vi "Dashboard Main.vi"() -> ()   [LabVIEW 2013]
uses:
  <vilib>/Rock Robotics/WPI/Camera/WPI_CameraSettings Read MJPG.ctl
  <vilib>/Rock Robotics/WPI/Camera/WPI_CameraImageSize.ctl
  <vilib>/Rock Robotics/WPI/Dashboard/WPI_DashboardLogging Global.vi
  <vilib>/vision/NI_Vision_Development_Module.lvlib
panel:
  out "Left":dbl(slide) scale=-1.0..1.0
  out "Right":dbl(slide) scale=-1.0..1.0
  out "Switch States":bool[](array[boolean])
  out "Catapult State":string
  out "Skeleton Detected":bool
  out "Right Triggered":bool
  out "Left Triggered":bool
  in  "Autonomous Mode":T1(ring)
  out "Right Speed":dbl(knob) scale=-11.0..11.0
  out "Left Speed":dbl(knob) scale=-11.0..11.0
  out "Teleop Time":dbl(slide) scale=0.0..150.0
  out "Right Power":dbl(slide) scale=-1.0..1.0
  out "Left Power":dbl(slide) scale=-1.0..1.0
  in  "Camera view range":dbl=33.5 format="%#_13g"
  out "Time Remaining":dbl(slide) scale=0.0..150.0
  in  "stop":bool
  out "Camera IP":string
  in  "DB Camera Config":bool
  out "Image Message":string="Timeout in Camera Communications"
  in  "Rec Mode":enum32{"Stop", "Record", "Playback"}(radio)
  out "Secondary Driver Camera":T2(plugin-control)
  out "Primary Driver Camera":T2(plugin-control)
  # "Primary Driver Side"
  # "Secondary Driver Side"
  # "TeleOperated"
  # "Autonomous"
  # "Checklist:\n1: DO WE HAVE A CHARGED BATTERY?\n2: Is the robot plugged in?\n3: Is the robot turned on?\n4: Are the ball(s) in the correct position?\n5: Set up Autonomous (One or Two balls?)"
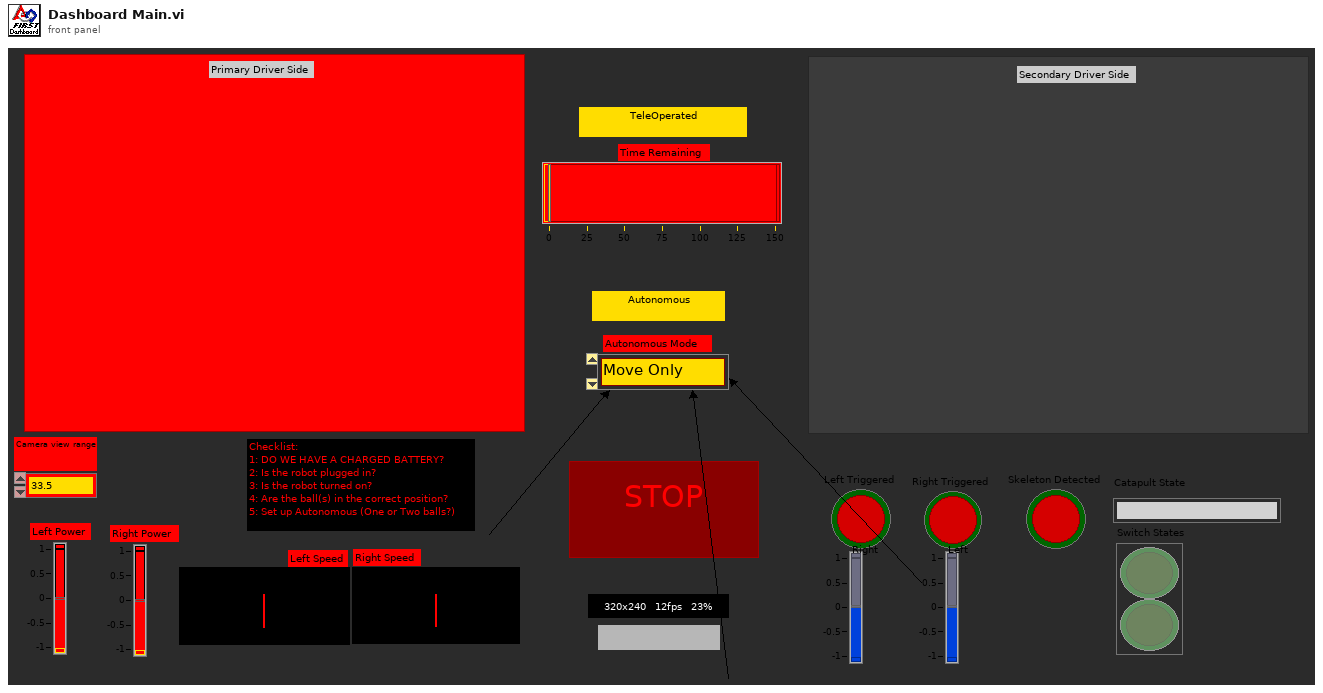
[diagram p1: front panel]
types:
  T1 = enum16{"Move Only", "One Ball", "Two Ball", "Three Ball", "Two Ball Hot", "One Ball Hot", "Nothing"}
  T2 = typedef "IMAQ Image.ctl" = refnum<image>
  T3 = typedef "Image Type" = u32
  T4 = cluster{"Left Power":dbl, "Right Power":dbl, "Shooter State":enum16{"Nothing", "Cocked", "Fire", "Load"}, "Loader State":enum16{"Loader Up", "Loader Down", "Ball In Possesion"}, "Auto Time":dbl, "Tele Time":dbl, "Driver":dbl, "Not Allowed":bool, "Right Speed":dbl, "Left Speed":dbl}
  T5 = cluster{"Digital Inputs":bool[], "Digital Outputs":bool[]}
  T6 = cluster{"Competition mode":bool, "Robot Link":bool, "Autonomous":bool, "Enabled":bool, "E-Stop":bool, "Simulated":bool, "TestMode":bool, "Docked Window":bool}
  T7 = typedef "Vector4.ctl" = cluster{"x":sgl, "y":sgl, "z":sgl, "w":sgl}
  T8 = typedef "SkeletonTrackState.ctl" = enum32{"NotTracked", "PositionOnly", "Tracked"}
  T9 = typedef "WPI_JoystickDeviceDataRaw.ctl" = cluster{"axis 1":i8, "axis 2":i8, "axis 3":i8, "axis 4":i8, "axis 5":i8, "axis 6":i8, "Buttons":u16}
  T10 = cluster{cluster{"Version String":string, "Number of Players":i8, "Flags":u32, "FloorClipPlane":T7, "Gravity Normal":cluster{"x":sgl, "y":sgl, "z":sgl}}, cluster{"TrackingState":u8[], "Overall Position":cluster{"x":sgl, "y":sgl, "z":sgl}, "Quality":u32, "TrackState":T8}, "Skeleton Vertices":cluster{"x":sgl, "y":sgl, "z":sgl}[], "Joystick":T9, "Joystick 2":T9, "Custom Data":string}
  T11 = typedef "WPI_CameraSettings Read MJPG.ctl" = cluster{"fps":i32, "compression":i32, "Image Size":T12}
  T12 = typedef "WPI_CameraImageSize.ctl" = enum16{"640x480", "320x240", "160x120"}
  T13 = cluster{"Left":i32, "Top":i32, "Right":i32, "Bottom":i32}
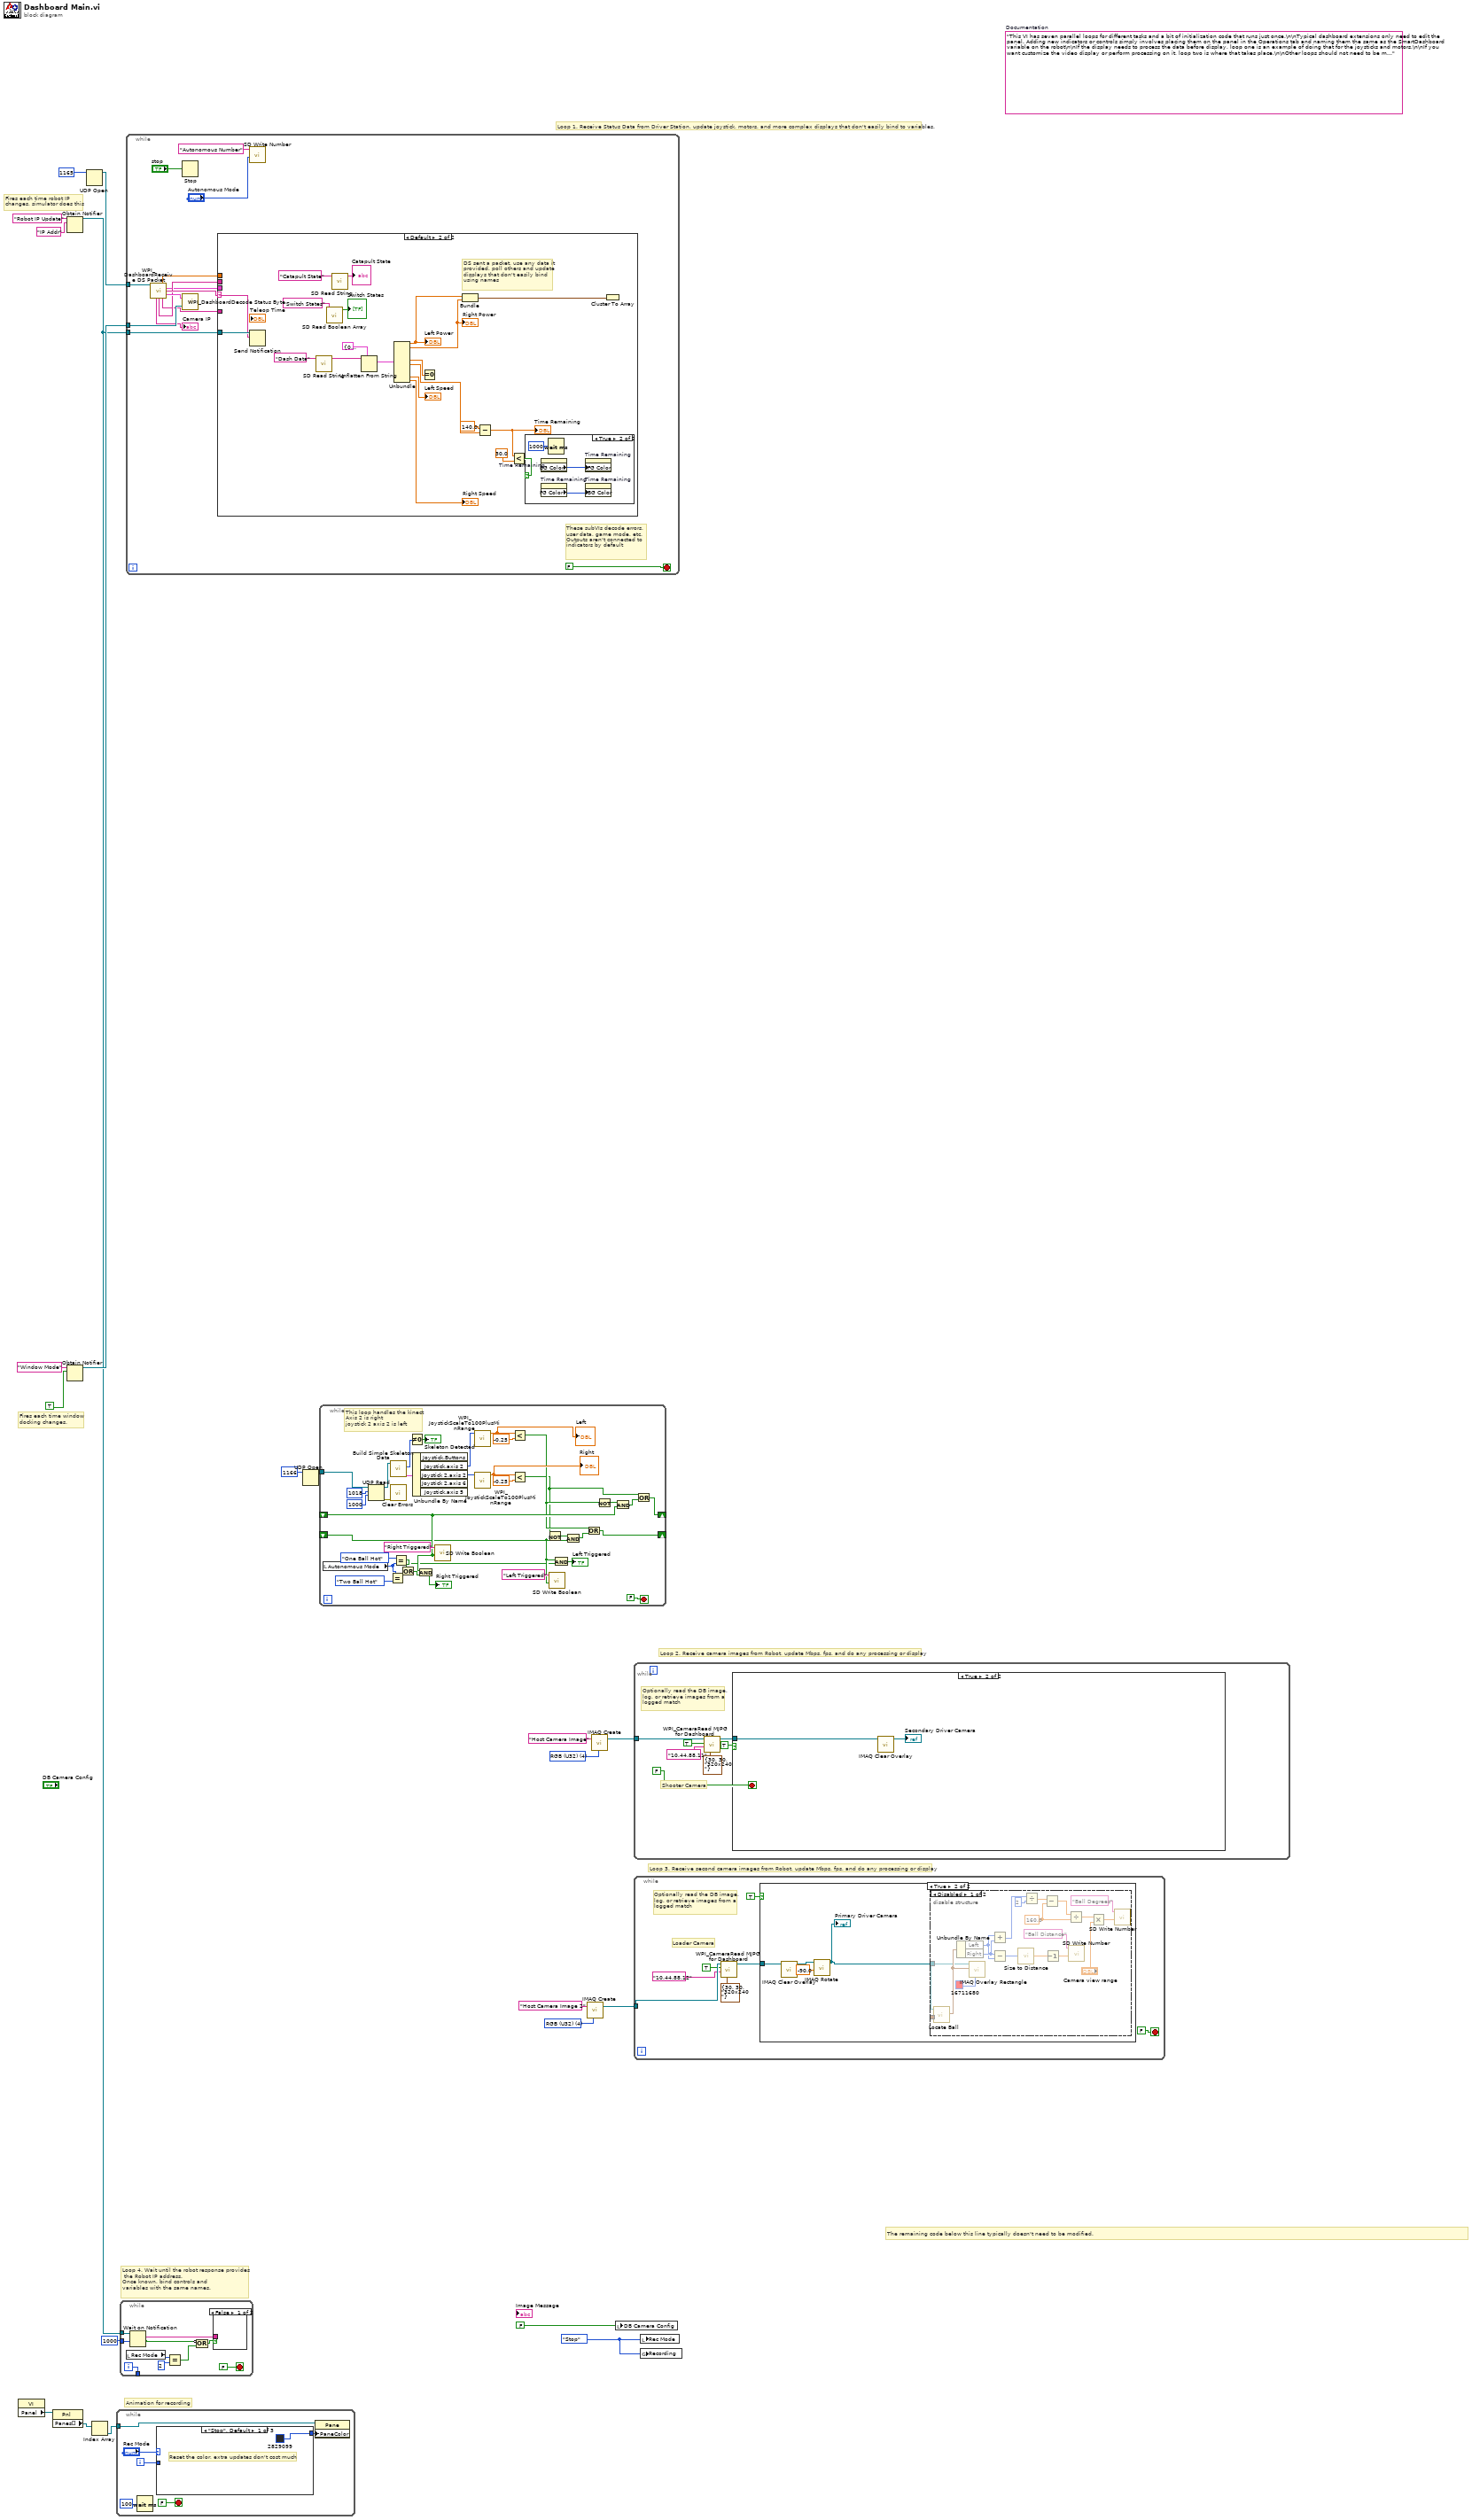
[diagram p0: block diagram]
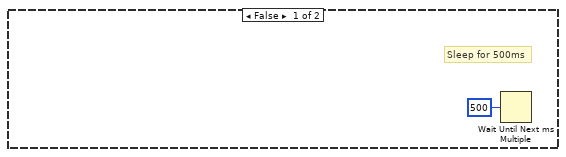
[diagram p2: hidden frame]
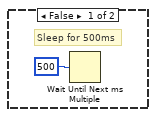
[diagram p3: hidden frame]
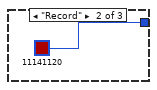
[diagram p5: hidden frame]
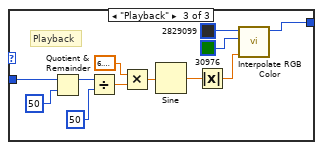
[diagram p6: hidden frame]
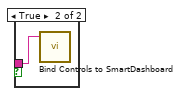
[diagram p7: hidden frame]
diagram:
  w5 = T3 4 items=["Grayscale (U8)", "Grayscale (I16)", "Grayscale (SGL)", "Complex (CSG)", "RGB (U32)", "HSL (U32)", "RGB (U64)"] ("Image Type")
  w6 = T3 4 items=["Grayscale (U8)", "Grayscale (I16)", "Grayscale (SGL)", "Complex (CSG)", "RGB (U32)", "HSL (U32)", "RGB (U64)"] ("Image Type")
  w10 = enum32{"Stop", "Record", "Playback"}."Stop" ("Rec Mode")
  (unwired) "This VI has seven parallel loops for different tasks and a bit of initialization code that runs just once.\n\nTypical dashboard extensions only need to edit the panel. Adding new indicators or controls simply involves placing them on the panel in the Operations tab and naming them the same as the SmartDashboard variable on the robot\n\nIf the display needs to process the data before display, loop one is an example of doing that for the joysticks and motors.\n\nIf you want customize the video display or perform processing on it, loop two is where that takes place.\n\nOther loops should not need to be modified. They are pretty standard, and document the task they perform."  # Documentation
  # "Loop 3. Receive second camera images from Robot, update Mbps, fps, and do any processing or display"
  # "Loop 2. Receive camera images from Robot, update Mbps, fps, and do any processing or display"
  # "Animation for recording"
  # "Fires each time robot IP\nchanges, simulator does this"
  # "Fires each time window\ndocking changes."
  # "The remaining code below this line typically doesn't need to be modified."
  # "Loop 4. Wait until the robot response provides\n the Robot IP address.\nOnce known, bind controls and\nvariables with the same names."
  # "Loop 1. Receive Status Data from Driver Station, update joystick, motors, and more complex displays that don't easily bind to variables."
  n1 = property class="VI"() -> ("Panel"=w14:refnum<vi>)  [unwired: 2 in, 2 out]
  n2 = property class="Pnl"(reference=w14) -> ("Panes[]"=w15:refnum<vi>[])  [unwired: 1 in, 2 out]
  n3 = Obtain Notifier(name (unnamed)="Robot IP Update", notification data type="IP Addr" ("name (unnamed)")) -> (notifier out=w9:refnum<notifier>)  [unwired: 2 in, 2 out]
  n4 = Obtain Notifier(name (unnamed)="Window Mode", notification data type=TRUE) -> (notifier out=w11:refnum<notifier>)  [unwired: 2 in, 2 out]
  n5 = UDP Open(11:u16 1165 ("port")) -> (port=w21:refnum<k16>)  [unwired: 2 in, 4 out]
  n6 = Index Array(array=w15) -> (element=w13:refnum<vi>)  [unwired: 1 in]
  n7 = while {
    tunnel: w13 -> [w24]
    i -> [w27]
    stop <- FALSE stop-if-true
    n8 = Wait (ms)(milliseconds to wait=u32 100) -> ()  [unwired: 1 out]
    n9 = case shown="\"Stop\", Default" "Rec Mode" {
      tunnel: w27 -> [_ _ w42]
      tunnel: [u32 2829099 ("Base Color") u32 11141120 ("Target Color") w31] -> w23
      frame "Stop", Default {
        # "Reset the color, extra updates don't cost much"
      }
      frame "Record" {
      }
      frame "Playback" {
        # "Playback"
        n10 = Quotient & Remainder(x=w42, y=u32 50 ("milliseconds to wait")) -> (x-y*floor(x/y)=w38:u32)  [unwired: 1 out]
        n11 = Divide(x=w38, y=u32 50 ("milliseconds to wait")) -> (x/y=w35:dbl)
        n12 = Multiply(x=6.283185307179586, y=w35) -> (x*y=w40:dbl)
        n13 = Sine(x=w40) -> (sin(x)=w39:dbl)
        n14 = Absolute Value(x=w39) -> (abs(x)=w32:dbl)
        n15 = call "Interpolate RGB Color.vi"("Proportion"=w32, "Target Color"=u32 30976, "Base Color"=u32 2829099) -> ("Result Color"=w31:u32)  [unwired: 8 in]
      }
    }
    n16 = property class="Pane"(reference=w24, "PaneColor"=w23) -> ()  [unwired: 1 in, 2 out]
  }
  n17 = while {
    tunnel: w9 -> [w51]
    tunnel: [w49] -> _
    tunnel: u32 1000 ("milliseconds to wait") -> [w48]
    i -> [w49]
    stop <- FALSE stop-if-true
    n18 = local read "Rec Mode"() -> (w44:enum32{"Stop", "Record", "Playback"})
    n19 = Wait on Notification(notifier=w51, timeout in ms (-1)=w48) -> (notification=w50:string, timed out?=w46:bool)  [unwired: 2 in, 2 out]
    n20 = Equal?(x=w44, y=u16 2 ("Rec Mode")) -> (x = y?=w45:bool)
    n21 = Compound Arithmetic op=OR(invert w46, w45) -> (w47:bool)
    n22 = case shown="False" w47 {
      tunnel: w50 -> [_ w53]
      frame False {
      }
      frame True {
        n23 = call <vilib>:"Bind Controls to SmartDashboard.vi"("Server IP Address"=w53) -> ()  [unwired: 11 in]
      }
    }
  }
  n24 = while {
    tunnel: w21 -> [w65]
    tunnel: w9 -> [w63]
    tunnel: w11 -> [w64]
    stop <- FALSE stop-if-true
    # "These subVIs decode errors, user data, game mode, etc.\nOutputs aren't connected to indicators by default"
    n25 = call <vilib>:"WPI_DashboardReceive DS Packet.vi"("Recv Socket"=w65) -> ("Battery"=w58:sgl, "Driver Station"=w59:T5, "Robot IP Address"=w62:string, "Status"=w66:T6, "Camera IP Address"=→"Camera IP":string, "Low Priority User Data"=w61:string, "High Priority User Data"=w60:string)  [unwired: 1 in, 7 out]
    n26 = Stop(stop? (T)="stop") -> ()
    n27 = call <vilib>:"WPI_DashboardDecode Status Byte.vi"("Window Mode Notifier"=w64, "Status"=w66) -> ()  [unwired: 2 out]
    n28 = case shown="Default" w62 {
      selector: w62 -> [_ w87]
      tunnel: w63 -> [_ w88]
      tunnel: w61 -> [_ _]
      tunnel: w60 -> [_ _]
      tunnel: w59 -> [_ _]
      tunnel: w58 -> [_ _]
      frame "0.0.0.0" {
        # "DS not sending packets, or no robot exists yet.\nDon't poll the variables"
      }
      frame Default {
        # "DS sent a packet. use any data it\nprovided, poll others and update\ndisplays that don't easily bind\nusing names"
        n29 = Send Notification(notification=w87, notifier=w88) -> ()  [unwired: 1 in, 2 out]
        n30 = call <vilib>:"SD Read String.vi"("Name"="Dash Data") -> ("String"=w84:string)  [unwired: 8 in, 2 out]
        n31 = call <vilib>:"SD Read Boolean Array.vi"("Name"="Switch States") -> ("Boolean Array"=→"Switch States":bool[])  [unwired: 8 in, 2 out]
        n32 = call <vilib>:"SD Read String.vi"("Name"="Catapult State") -> ("String"=→"Catapult State":string)  [unwired: 8 in, 2 out]
        n33 = Unflatten From String(type=T4 {"Left Power"=0.0, "Right Power"=0.0, "Shooter State"=enum."Nothing", "Loader State"=enum."Loader Up", "Auto Time"=0.0, "Tele Time"=0.0, "Driver"=0.0, "Not Allowed"=FALSE, "Right Speed"=0.0, "Left Speed"=0.0} ("To Dashboard"), binary string=w84) -> (value=w83:T4)  [unwired: 3 in, 2 out]
        n34 = Unbundle(w83) -> ("Left Power"=w76:dbl, "Right Power"=w75:dbl, "Auto Time"=w81:dbl, "Tele Time"=w82:dbl, "Right Speed"=→"Left Speed":dbl, "Left Speed"=→"Right Speed":dbl)  [unwired: 4 out]
        "Left Power" <- w76
        "Right Power" <- w75
        n35 = Equal To 0?(x=w81) -> ()  [unwired: 1 out]
        n36 = Bundle("Left Power"=w76, "Right Power"=w75) -> (w80:cluster{"Left Power":dbl, "Right Power":dbl})  [unwired: 1 in]
        n37 = Subtract(x=140.0, y=w82) -> (x-y=w74:dbl)
        "Time Remaining" <- w74
        n38 = Less?(x=w74, y=30.0 ("x")) -> (x < y?=w72:bool)
        n39 = case shown="True" w72 {
          frame False {
          }
          frame True {
            n40 = property on="Time Remaining" class="Slide (strict)"() -> ("BG Color"=w90:u32)  [unwired: 2 in, 2 out]
            n41 = property on="Time Remaining" class="Slide (strict)"() -> ("FG Color"=w91:u32)  [unwired: 2 in, 2 out]
            n42 = Wait (ms)(milliseconds to wait=u32 1000) -> ()  [unwired: 1 out]
            n43 = property on="Time Remaining" class="Slide (strict)"("FG Color"=w90) -> ()  [unwired: 2 in, 2 out]
            n44 = property on="Time Remaining" class="Slide (strict)"("BG Color"=w91) -> ()  [unwired: 2 in, 2 out]
          }
        }
        n45 = Cluster To Array(cluster=w80) -> ()  [unwired: 1 out]
      }
    }
    n46 = call <vilib>:"SD Write Number.vi"("Numeric"="Autonomous Mode", "Name"="Autonomous Number") -> ()  [unwired: 8 in, 2 out]
  }
  n47 = UDP Open(11:u16 1166 ("port")) -> (port=w1:refnum<k16>)  [unwired: 2 in, 4 out]
  n48 = while {
    tunnel: w1 -> [w124]
    shift-right: [w107] -> _
    shift-left: _ -> [w103]
    shift-right: [w111] -> _
    shift-left: _ -> [w101]
    stop <- FALSE stop-if-true
    # "This loop handles the kinect\nAxis 2 is right\njoystick 2 axis 2 is left"
    n49 = local read "Autonomous Mode"() -> (w99:T1)
    n50 = UDP Read(connection ID=w124, max size (548)=1018 ("bytes to read"), timeout ms (25000)=1000) -> (error out=w120:errorcluster, 3:w117:refnum<k16>)  [unwired: 1 in, 3 out]
    n51 = Equal?(x=w99, y=T1."Two Ball Hot") -> (x = y?=w96:bool)
    n52 = call "Build Simple Skeleton Data.vi"("connection ID"=w117) -> ("Kinect Outputs"=w122:T10, "NumPlayers"=w123:i8)  [unwired: 6 in, 3 out]
    n53 = call <vilib>:"Clear Errors.vi"("error in (no error)"=w120) -> ()  [unwired: 6 in, 1 out]
    n54 = Equal?(x=T1."One Ball Hot", y=w99) -> (x = y?=w97:bool)
    n55 = Or(x=w97, y=w96) -> (x .or. y?=w95:bool)
    n56 = Not Equal To 0?(x=w123) -> (x != 0?=→"Skeleton Detected":bool)
    n57 = Unbundle By Name(w122) -> ("Joystick.axis 2"=w119:i8, "Joystick 2.axis 2"=w118:i8)  [unwired: 3 out]
    n58 = And(x=w103, y=w95) -> (x .and. y?=→"Right Triggered":bool)
    n59 = call <vilib>:"SD Write Boolean.vi"("Boolean"=w103, "Name"="Right Triggered") -> ()  [unwired: 8 in, 2 out]
    n60 = call <vilib>:"WPI_JoystickScaleTo100PlusMinRange.vi"("RawValue"=w119) -> ("ScaledToPercentRange"=w94:dbl)  [unwired: 1 in, 9 out]
    "Left" <- w94
    n61 = call <vilib>:"WPI_JoystickScaleTo100PlusMinRange.vi"("RawValue"=w118) -> ("ScaledToPercentRange"=w113:dbl)  [unwired: 1 in, 9 out]
    "Right" <- w113
    n62 = Less?(x=w94, y=-0.25) -> (x < y?=w93:bool)
    n63 = Less?(x=w113, y=-0.25 ("x")) -> (x < y?=w92:bool)
    n64 = Not(x=w92) -> (.not. x?=w110:bool)
    n65 = call <vilib>:"SD Write Boolean.vi"("Boolean"=w101, "Name"="Left Triggered") -> ()  [unwired: 8 in, 2 out]
    n66 = And(x=w101, y=w95) -> (x .and. y?=→"Left Triggered":bool)
    n67 = And(x=w110, y=w101) -> (x .and. y?=w112:bool)
    n68 = Or(x=w93, y=w112) -> (x .or. y?=w111:bool)
    n69 = Not(x=w93) -> (.not. x?=w109:bool)
    n70 = And(x=w109, y=w103) -> (x .and. y?=w108:bool)
    n71 = Or(x=w92, y=w108) -> (x .or. y?=w107:bool)
  }
  n72 = call "IMAQ Create"("Image Name"="Host Camera Image 2", "Image Type"=w6) -> ("New Image"=w8:T2)  [unwired: 2 in, 2 out]
  n73 = call "IMAQ Create"("Image Name"="Host Camera Image", "Image Type"=w5) -> ("New Image"=w3:T2)  [unwired: 2 in, 2 out]
  n74 = local write "DB Camera Config"(FALSE ("Visible")) -> ()
  n75 = while {
    tunnel: w8 -> [w132]
    stop <- FALSE stop-if-true
    # "Loader Camera"
    # "Optionally read the DB image,\nlog, or retrieve images from a\nlogged match"
    n76 = call <vilib>:"WPI_CameraRead MJPG for Dashboard.vi"("Camera Settings"=T11 {"fps"=30, "compression"=30, "Image Size"=enum."320x240"}, "Camera IP"="10.44.88.12", "Enable"=TRUE ("Enable 2"), "Refnum in"=w132) -> ("Refnum out"=w131:T2)  [unwired: 4 in, 3 out]
    n77 = case shown="True" TRUE ("Enable 2") {
      tunnel: w131 -> [_ w138]
      frame False {
        # "Sleep for 500ms"
        n78 = Wait Until Next ms Multiple(millisecond multiple=u32 500) -> ()  [unwired: 1 out]
      }
      frame True {
        n79 = call "IMAQ Clear Overlay"("Image"=w138) -> ("Image Out"=w135:T2)  [unwired: 2 in, 8 out]
        n80 = call "IMAQ Rotate"("Angle (degrees)"=sgl -90.0, "Image Src"=w135) -> ("Image Dst Out"=w136:T2)  [unwired: 8 in, 1 out]
        "Primary Driver Camera" <- w136
        n81 = disable-structure shown="Disabled" {
          disable-tunnel: w136 -> [w141 _]
          disable-tunnel: _ -> [w140 _]
          frame Disabled {
            w153 = 160.0 ("y")
            n82 = call "Locate Ball.vi"("New Image"=w141, "Hue Selector"=w140) -> ("Rectangle"=w147:T13)  [unwired: 7 in, 1 out]
            n83 = Unbundle By Name(w147) -> ("Left"=w149:i32, "Right"=w150:i32)
            n84 = call "IMAQ Overlay Rectangle"("Color"=u32 16711680, "Rectangle"=w147, "Image"=w141) -> ()  [unwired: 7 in, 2 out]
            n85 = Add(x=w149, y=w150) -> (x+y=w157:i32)
            n86 = Subtract(x=w150, y=w149) -> (x-y=w144:i32)
            n87 = call "Size to Distance.vi"("Numeric"=w144) -> ("Numeric 2"=w143:dbl)
            n88 = Divide(x=w157, y=2) -> (x/y=w155:dbl)
            n89 = Subtract(x=w155, y=w153) -> (x-y=w154:dbl)
            n90 = Decrement(x=w143) -> (x-1=w142:dbl)
            n91 = Divide(x=w154, y=w153) -> (x/y=w152:dbl)
            n92 = call <vilib>:"SD Write Number.vi"("Numeric"=w142, "Name"="Ball Distance") -> ()  [unwired: 8 in, 2 out]
            n93 = Multiply(x=w152, y="Camera view range") -> (x*y=w145:dbl)
            n94 = call <vilib>:"SD Write Number.vi"("Numeric"=w145, "Name"="Ball Degrees") -> ()  [unwired: 8 in, 2 out]
          }
          frame Enabled {
          }
        }
      }
    }
  }
  n95 = while {
    tunnel: w3 -> [w163]
    stop <- FALSE stop-if-true
    # "Shooter Camera"
    # "Optionally read the DB image,\nlog, or retrieve images from a\nlogged match"
    n96 = call <vilib>:"WPI_CameraRead MJPG for Dashboard.vi"("Camera Settings"=T11 {"fps"=30, "compression"=30, "Image Size"=enum."320x240"}, "Camera IP"="10.44.88.11", "Enable"=TRUE ("Enable 2"), "Refnum in"=w163) -> ("Refnum out"=w162:T2)  [unwired: 4 in, 3 out]
    n97 = case shown="True" TRUE ("Enable 2") {
      tunnel: w162 -> [_ w167]
      frame False {
        # "Sleep for 500ms"
        n98 = Wait Until Next ms Multiple(millisecond multiple=u32 500) -> ()  [unwired: 1 out]
      }
      frame True {
        n99 = call "IMAQ Clear Overlay"("Image"=w167) -> ("Image Out"=→"Secondary Driver Camera":T2)  [unwired: 2 in, 8 out]
      }
    }
  }
  n100 = local write "Rec Mode"(w10) -> ()
  n101 = global write "WPI_DashboardLogging Global.vi" "Recording"(w10) -> ()
